vi "Command.vi"(7 "receive data (true)":bool=TRUE, 8 "error in (no error)":errorcluster, 9 "parameters":string[](array[string]), 10 "command":string, 11 "VGC in":refnum<class "PL Inficon VGC.lvclass">) -> (0 "error out":errorcluster, 2 "response data":string[](array[string]), 3 "VGC out":refnum<class "PL Inficon VGC.lvclass">)   [LabVIEW 2015, in "PL Inficon VGC.lvclass"]
doc: "Sends <b>command</b> with <b>parameters</b> to device and returns <b>response data</b> if necessary."
uses:
  PL Inficon VGC.lvclass
  PL Inficon VGC.lvclass/PL Inficon VGC.ctl
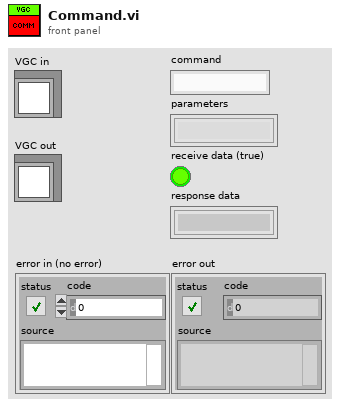
[diagram p1: front panel]
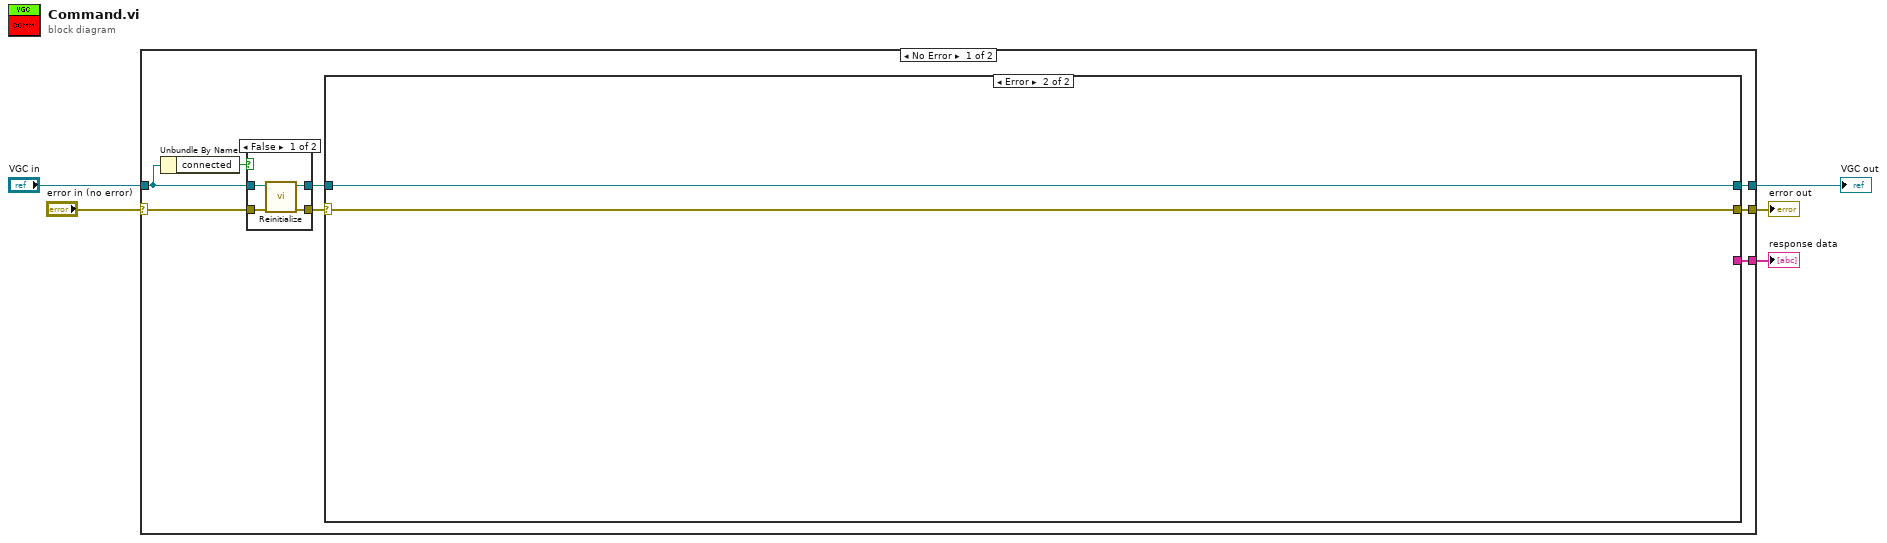
[diagram p0: block diagram]
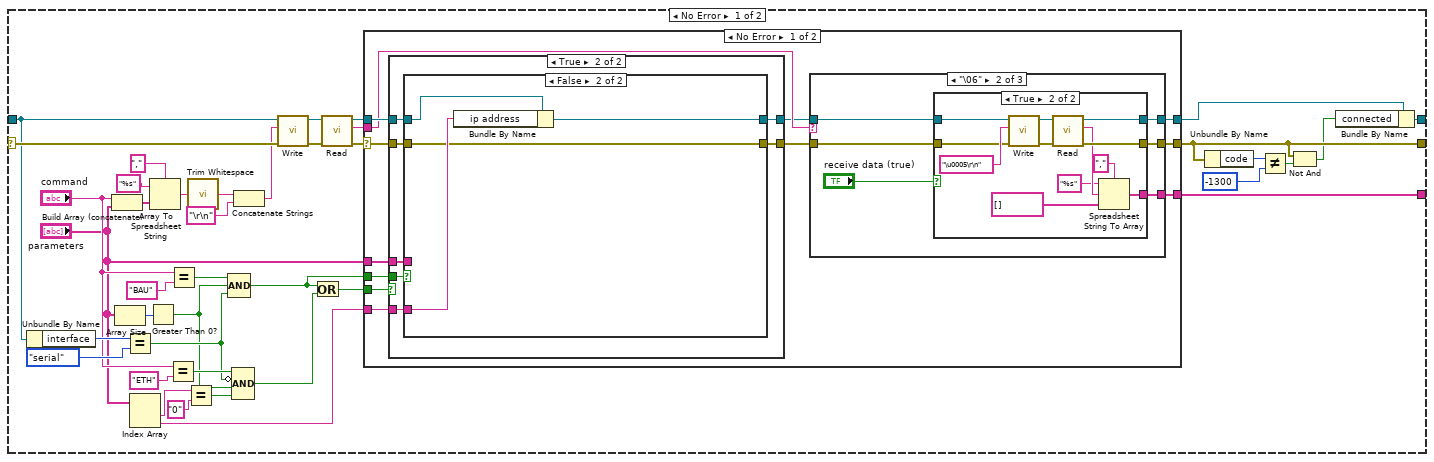
[diagram p2: hidden frame]
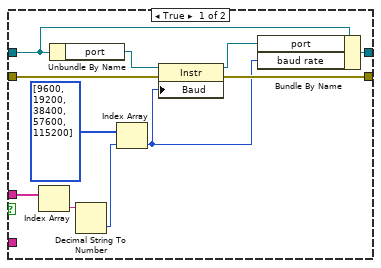
[diagram p4: hidden frame]
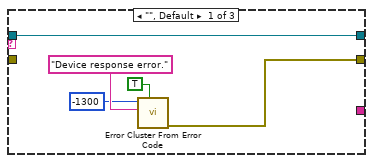
[diagram p5: hidden frame]
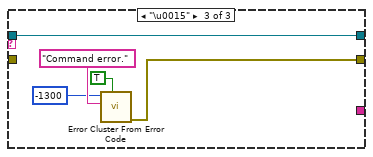
[diagram p7: hidden frame]
diagram:
  n1 = case shown="No Error" "error in (no error)" {
    selector: "error in (no error)" -> [w11 w131]
    tunnel: "VGC in" -> [w12 w130]
    tunnel: [w8 w131] -> w1
    tunnel: [w7 w130] -> w3
    tunnel: [w6 _] -> w2
    frame No Error {
      n2 = Unbundle By Name(w12) -> ("connected"=w13:bool)
      n3 = case shown="False" w13 {
        tunnel: w12 -> [w127 w129]
        tunnel: w11 -> [w126 w128]
        tunnel: [w125 w129] -> w9
        tunnel: [w124 w128] -> w10
        frame False {
          n4 = call "Reinitialize.vi"("error in (no error)"=w126, "VGC in"=w127) -> ("error out"=w124:errorcluster, "VGC out"=w125:refnum<class "PL Inficon VGC.lvclass">)  [unwired: 8 in]
        }
        frame True {
        }
      }
      n5 = case shown="Error" w10 {
        selector: w10 -> [w53 w123]
        tunnel: w9 -> [w44 w122]
        tunnel: [w30 w123] -> w8
        tunnel: [w28 w122] -> w7
        tunnel: [w46 _] -> w6
        frame No Error {
          n6 = Unbundle By Name(w44) -> ("interface"=w43:enum16{"serial", "network"})
          n7 = Build Array (concatenate)("command", "parameters") -> (w52:string[])
          n8 = Array Size(array="parameters") -> (size(s)=w39:i32)
          n9 = Equal?(x=w43, y=enum16{"serial", "network"}."serial") -> (x = y?=w21:bool)
          n10 = Index Array(array="parameters") -> (element #1=w18:string, element #2=w14:string)  [unwired: 2 in]
          n11 = Greater Than 0?(x=w39) -> (x > 0?=w20:bool)
          n12 = Array To Spreadsheet String(delimiter (Tab)=",", array=w52, 3:"%s" ("format string")) -> (spreadsheet string=w49:string)
          n13 = Equal?(x="command", y="ETH") -> (x = y?=w22:bool)
          n14 = Equal?(x="command", y="BAU") -> (x = y?=w40:bool)
          n15 = Equal?(x=w18, y="0") -> (x = y?=w16:bool)
          n16 = call <vilib>:"Trim Whitespace.vi"("string"=w49) -> ("trimmed string"=w45:string)  [unwired: 1 in]
          n17 = Compound Arithmetic op=AND(w40, w20, w21) -> (w25:bool)
          n18 = Compound Arithmetic op=AND(w22, invert w21, w20, w16) -> (w15:bool)
          n19 = Concatenate Strings(w45, "\r\n" ("string")) -> (w47:string)
          n20 = call "Write.vi"("error in (no error)"=w53, "write buffer"=w47, "VGC in"=w44) -> ("error out"=w37:errorcluster, "VGC out"=w38:refnum<class "PL Inficon VGC.lvclass">)  [unwired: 7 in]
          n21 = Or(x=w25, y=w15) -> (x .or. y?=w26:bool)
          n22 = call "Read.vi"("error in (no error)"=w37, "VGC in"=w38) -> ("error out"=w35:errorcluster, "read buffer"=w36:string, "VGC out"=w34:refnum<class "PL Inficon VGC.lvclass">)  [unwired: 7 in]
          n23 = case shown="No Error" w35 {
            selector: w35 -> [w61 w120]
            tunnel: w34 -> [w62 w121]
            tunnel: [w65 w121] -> w27
            tunnel: [w64 w120] -> w30
            tunnel: [w63 _] -> w46
            tunnel: w36 -> [w60 _]
            tunnel: "parameters" -> [w57 _]
            tunnel: w26 -> [w56 _]
            tunnel: w25 -> [w55 _]
            tunnel: w14 -> [w54 _]
            frame No Error {
              n24 = case shown="True" w56 {
                tunnel: w62 -> [w67 w72]
                tunnel: [w67 w71] -> w59
                tunnel: [w66 w70] -> w58
                tunnel: w61 -> [w66 w73]
                tunnel: w57 -> [_ w74]
                tunnel: w55 -> [_ w69]
                tunnel: w54 -> [_ w68]
                frame False {
                }
                frame True {
                  n25 = case shown="False" w69 {
                    tunnel: w74 -> [w85 _]
                    tunnel: w73 -> [w80 w86]
                    tunnel: w72 -> [w79 w88]
                    tunnel: [w78 w89] -> w71
                    tunnel: [w76 w86] -> w70
                    tunnel: w68 -> [_ w87]
                    frame True {
                      n26 = Index Array(array=w85) -> (element=w82:string)  [unwired: 1 in]
                      n27 = Unbundle By Name(w79) -> ("port"=w81:refnum<visa-resource-name>)
                      n28 = Decimal String To Number(string=w82) -> (number=w83:i32)  [unwired: 2 in, 1 out]
                      n29 = Index Array(array=u32[] [9600, 19200, 38400, 57600, 115200], index=w83) -> (element=w75:u32)
                      n30 = property class="Instr"(reference=w81, error in=w80, "Baud"=w75) -> (reference out=w77:refnum<visa-resource-name>, error out=w76:errorcluster)
                      n31 = Bundle By Name(cluster=w79, "port"=w77, "baud rate"=w75) -> (w78:refnum<class "PL Inficon VGC.lvclass">)
                    }
                    frame False {
                      n32 = Bundle By Name(cluster=w88, "ip address"=w87) -> (w89:refnum<class "PL Inficon VGC.lvclass">)
                    }
                  }
                }
              }
              n33 = case shown="\"\\06\"" w60 {
                tunnel: w59 -> [w91 w100 w115]
                tunnel: [w91 w98 w115] -> w65
                tunnel: [w90 w96 w116] -> w64
                tunnel: w58 -> [_ w97 _]
                tunnel: [_ w95 _] -> w63
                frame "", Default {
                  n34 = call <vilib>:"Error Cluster From Error Code.vi"("show call chain? (False)"=TRUE, "error message (\"\")"="Device response error." ("format string"), "error code (0)"=-1300) -> ("error out"=w90:errorcluster)  [unwired: 6 in]
                }
                frame "\u0006" {
                  n35 = case shown="True" "receive data (true)" {
                    tunnel: w100 -> [w102 w114]
                    tunnel: [w102 w108] -> w98
                    tunnel: w97 -> [w101 w112]
                    tunnel: [w101 w109] -> w96
                    tunnel: [_ w103] -> w95
                    frame False {
                    }
                    frame True {
                      n36 = call "Write.vi"("error in (no error)"=w112, "write buffer"="\u0005\r\n", "VGC in"=w114) -> ("error out"=w110:errorcluster, "VGC out"=w111:refnum<class "PL Inficon VGC.lvclass">)  [unwired: 7 in]
                      n37 = call "Read.vi"("error in (no error)"=w110, "VGC in"=w111) -> ("error out"=w109:errorcluster, "read buffer"=w107:string, "VGC out"=w108:refnum<class "PL Inficon VGC.lvclass">)  [unwired: 7 in]
                      n38 = Spreadsheet String To Array(delimiter (Tab)=",", format string="%s", spreadsheet string=w107, array type (2D Dbl)=string[] []) -> (array=w103:string[])
                    }
                  }
                }
                frame "\u0015" {
                  n39 = call <vilib>:"Error Cluster From Error Code.vi"("show call chain? (False)"=TRUE, "error message (\"\")"="Command error." ("format string"), "error code (0)"=-1300) -> ("error out"=w116:errorcluster)  [unwired: 6 in]
                }
              }
            }
            frame Error {
            }
          }
          n40 = Unbundle By Name(w30) -> ("code"=w32:i32)
          n41 = Not Equal?(x=w32, y=-1300 ("error code (0)")) -> (x != y?=w33:bool)
          n42 = Not And(1:w33, 2:w30) -> (0:w29:bool)
          n43 = Bundle By Name(cluster=w27, "connected"=w29) -> (w28:refnum<class "PL Inficon VGC.lvclass">)
        }
        frame Error {
        }
      }
    }
    frame Error {
    }
  }
  "VGC out" <- w3
  "error out" <- w1
  "response data" <- w2
